vi "MRC Console Write Line.vi"(8 "error in (no error)":errorcluster, 11 "line":T1) -> (0 "error out":errorcluster)   [LabVIEW 2026, in "MrcLib.lvlib"]
doc: "MRC_Status MRC_CALLCONV MRC_Console_WriteLine(const struct MRC_String* line);"
uses:
  MrcLib.lvlib
  Types/MRC String.ctl
  MrcLib.dll
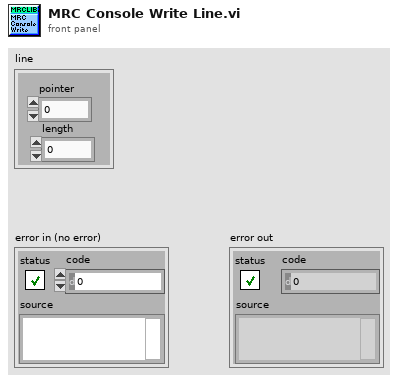
[diagram p1: front panel]
types:
  T1 = typedef "MRC String.ctl" = cluster{"pointer":u64, "length":u64}
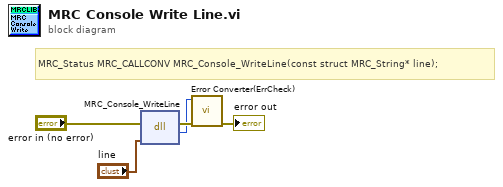
[diagram p0: block diagram]
diagram:
  # "MRC_Status MRC_CALLCONV MRC_Console_WriteLine(const struct MRC_String* line);"
  n1 = dll-call lib="MrcLib.*" fn="MRC_Console_WriteLine"(error in="error in (no error)", "line"="line") -> (error out=w2:errorcluster, "return type"=w1:i32)  [unwired: 3 in, 1 out]
  n2 = call "Error Converter(ErrCheck).vi"("error in (no error)"=w2, "status"=w1) -> ("error out"=→"error out":errorcluster)  [unwired: 9 in]
